vi "WriteDac_2.vi"(4 "ref":dbl=666.0, 5 "error in (no error)":errorcluster, 6 "value":dbl=666.0, 7 "mode":i32=1, 8 "DAC number":i32=1, 9 "Board address":i32=4660 format="%x") -> (0 "error out":errorcluster)   [LabVIEW 2011]
doc: "This VI is a wrapper for the \"tio32_WriteDac\" VI by LPSE. Its purpose is to increment the \"DAC number\" variable by 1, since the enum control for DAC number gives values 0-3 but the LPSE VI requires values 1-4. In addition, this VI converts the DAC number and voltage values into strings and outputs them to the global string variable used to populate the \"TI Debug Window\" VI."
uses:
  INA231/Global Variables.vi
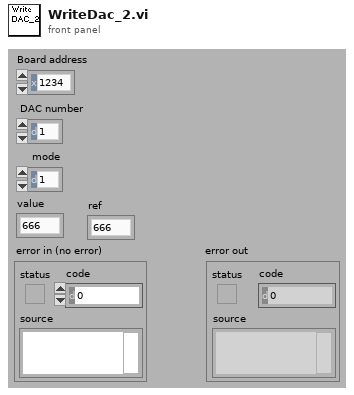
[diagram p1: front panel]
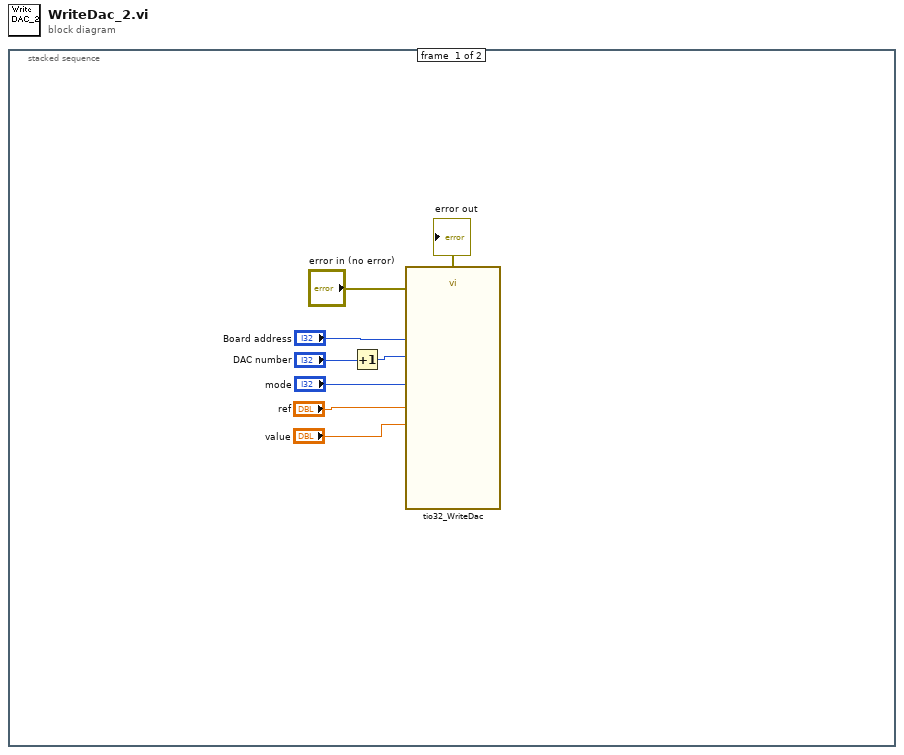
[diagram p0: block diagram]
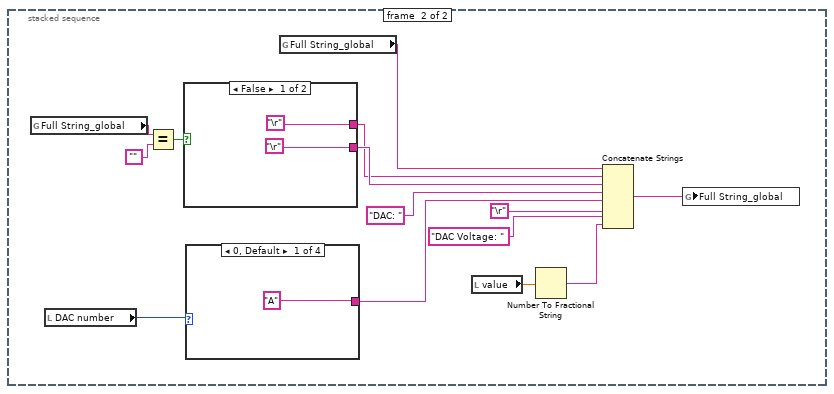
[diagram p2: hidden frame]
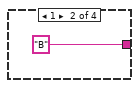
[diagram p3: hidden frame]
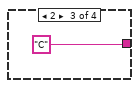
[diagram p4: hidden frame]
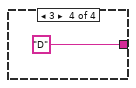
[diagram p5: hidden frame]
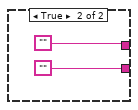
[diagram p6: hidden frame]
diagram:
  n1 = stacked-sequence {
    frame #0 {
      n2 = Increment(x="DAC number") -> (x+1=w2:i32)
      n3 = call "tio32_WriteDac.vi"("Board address"="Board address", "DAC number"=w2, "mode"="mode", "error in (no error)"="error in (no error)", "value"="value", "User Ref"="ref") -> ("error out"=→"error out":errorcluster)  [unwired: 7 in, 2 out]
    }
    frame #1 {
      n4 = global read "Global Variables.vi" "Full String_global"() -> (w15:string)
      n5 = local read "DAC number"() -> (w13:i32)
      n6 = Equal?(x=w15, y="") -> (x = y?=w14:bool)
      n7 = case shown="False" w14 {
        tunnel: ["\r" ""] -> w19
        tunnel: ["\r" ""] -> w20
        frame False {
        }
        frame True {
        }
      }
      n8 = case shown="0, Default" w13 {
        tunnel: ["A" "B" "C" "D"] -> w12
        frame 0, Default {
        }
        frame 1 {
        }
        frame 2 {
        }
        frame 3 {
        }
      }
      n9 = global read "Global Variables.vi" "Full String_global"() -> (w18:string)
      n10 = local read "value"() -> (w10:dbl)
      n11 = Number To Fractional String(number=w10) -> (F-format string=w9:string)  [unwired: 3 in]
      n12 = Concatenate Strings(w18, w19, w20, "DAC: ", w12, "\r", "DAC Voltage: ", w9) -> (w17:string)
      n13 = global write "Global Variables.vi" "Full String_global"(w17) -> ()
    }
  }
